vi "RDS Child Subscription.vi"(8 "error in (no error)":errorcluster, 11 "RDS Test Child in":refnum<class "RDS Test Child.lvclass">) -> (0 "error out":errorcluster, 2 "Subscribed IDs":T1[](array[typedef]), 3 "RDS Test Child out":refnum<class "RDS Test Child.lvclass">)   [LabVIEW 2015, in "RDS Test Child.lvlib" / "RDS Test Child.lvclass"]
uses:
  RDS Test Child.lvclass
  Libraries/RDS Framework/RDS Message ID.ctl
  RDS Parent Actor/RDS Parent Actor/RDS Parent Actor.lvclass/RDS Parent Actor.ctl
  RDS Parent Actor/RDS Parent Actor/RDS Parent Actor.lvclass
  Libraries/RDS Child Messages/RDS Child Messages.lvlib
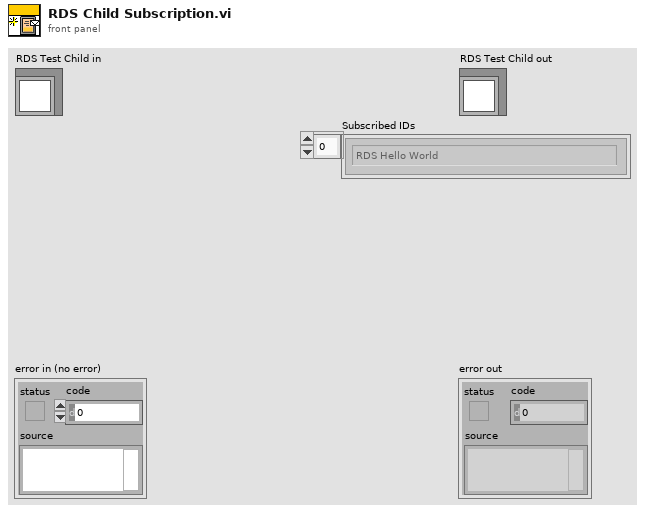
[diagram p1: front panel]
types:
  T1 = typedef "RDS Child Messages.lvlib/RDS Message ID.ctl" = enum16{"RDS Hello World", "String Message", "AIP_Status", "AIP_Command", "GPS_Data", "MCB_Command", "MCB_Status", "Compass_Data", "Depth_Data", "Battery_Data", "Contoller_State", "Set_Mag_Dev", "BTB_Shutdown", "State_Sample_Request", "State_Sample", "PID_Gains_Set", "Helm_Limiter_Set", "Helm_Heading_Command", "Helm_Steering_Command", "Helm_Status", "Controller_Message", "AIP_Set_Min_Depth", "Mission_Controller_State", "Mission_Upload", "Mission_Set_Op_and_Run", "Mission_Settings_Set"}
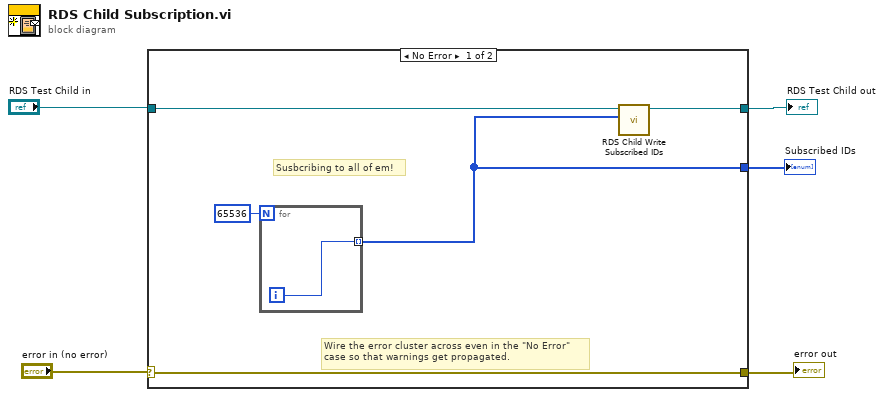
[diagram p0: block diagram]
diagram:
  n1 = case shown="No Error" "error in (no error)" {
    selector: "error in (no error)" -> [w10 w13]
    tunnel: [w10 w13] -> w4
    tunnel: [w8 w12] -> w3
    tunnel: "RDS Test Child in" -> [w9 w12]
    tunnel: [w6 _] -> w1
    frame No Error {
      # "Susbcribing to all of em!"
      # "Wire the error cluster across even in the \"No Error\"\ncase so that warnings get propagated."
      n2 = for {
        N: 65536 -> [_]
        tunnel: [w11] -> w6 mode=indexing
        i -> [w11]
      }
      n3 = call "RDS Child Write Subscribed IDs.vi"("Subscribed IDs"=w6, "RDS Parent Actor in"=w9) -> ("RDS Parent Actor out"=w8:refnum<class "RDS Test Child.lvclass">)  [unwired: 8 in, 1 out]
    }
    frame Error {
    }
  }
  "error out" <- w4
  "RDS Test Child out" <- w3
  "Subscribed IDs" <- w1
